vi "TCP单点接收.main.vi"(0 "IP地址":string="127.0.0.1" caption="服务名称", 1 "端口号":i32=6314, 2 "储存路径":path=path "D:/AA", 5 "error IO":errorcluster caption="错误输入") -> (14 "已收百分比":string, 15 "运行指示灯":bool, 19 "错误输出 2":errorcluster caption="错误输出")   [LabVIEW 2016, in "TCP文件传输系统.lvlib" / "TCP接收文件.lvlib"]
panel:
  in  "分一包（兆）":i64=40
  out "文件名":string
  out "2":errorcluster caption="错误输出"
  out "单包大小":i32
  out "帧数":i32
  out "帧号":i32
  out "错误输出":errorcluster
  out "路径 2":path
  out "已收次数":i32
  out "需接收次数":i32
  in  "停止 2":bool
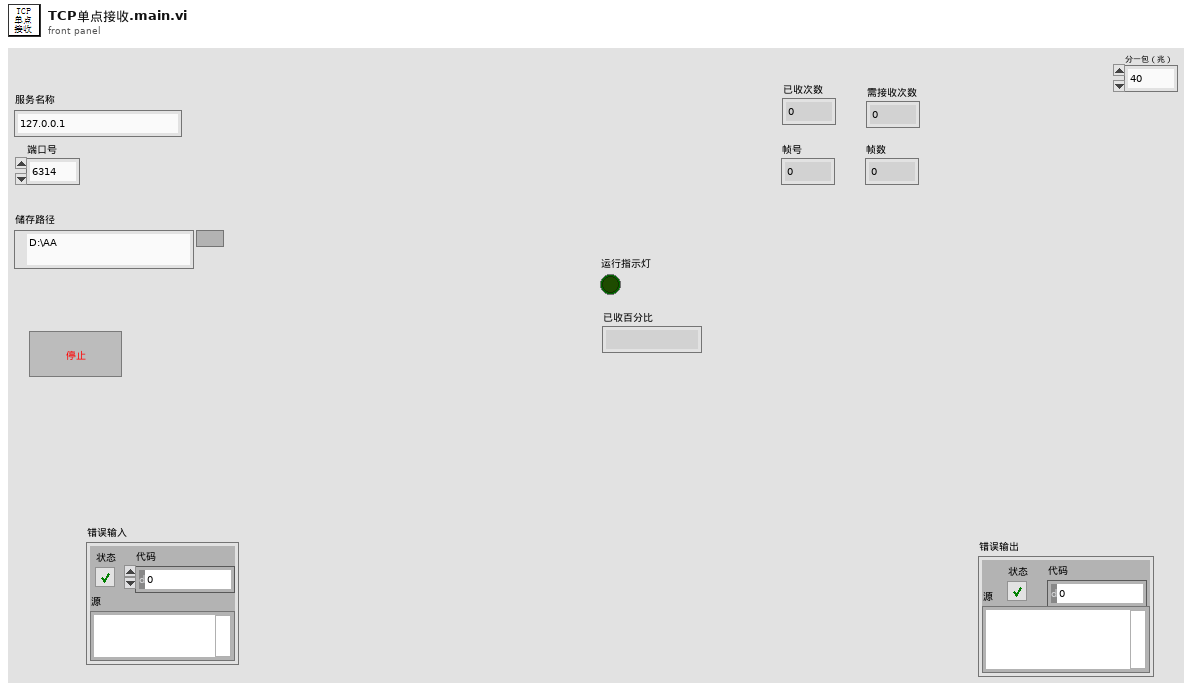
[diagram p1: front panel]
types:
  T1 = cluster{"网络灯":bool, "接收中":bool, "已接收百分比":string, "接收成功次数":dbl}
  T2 = enum16{"open", "replace", "create", "open or create", "replace or create", "replace or create with confirmation"}
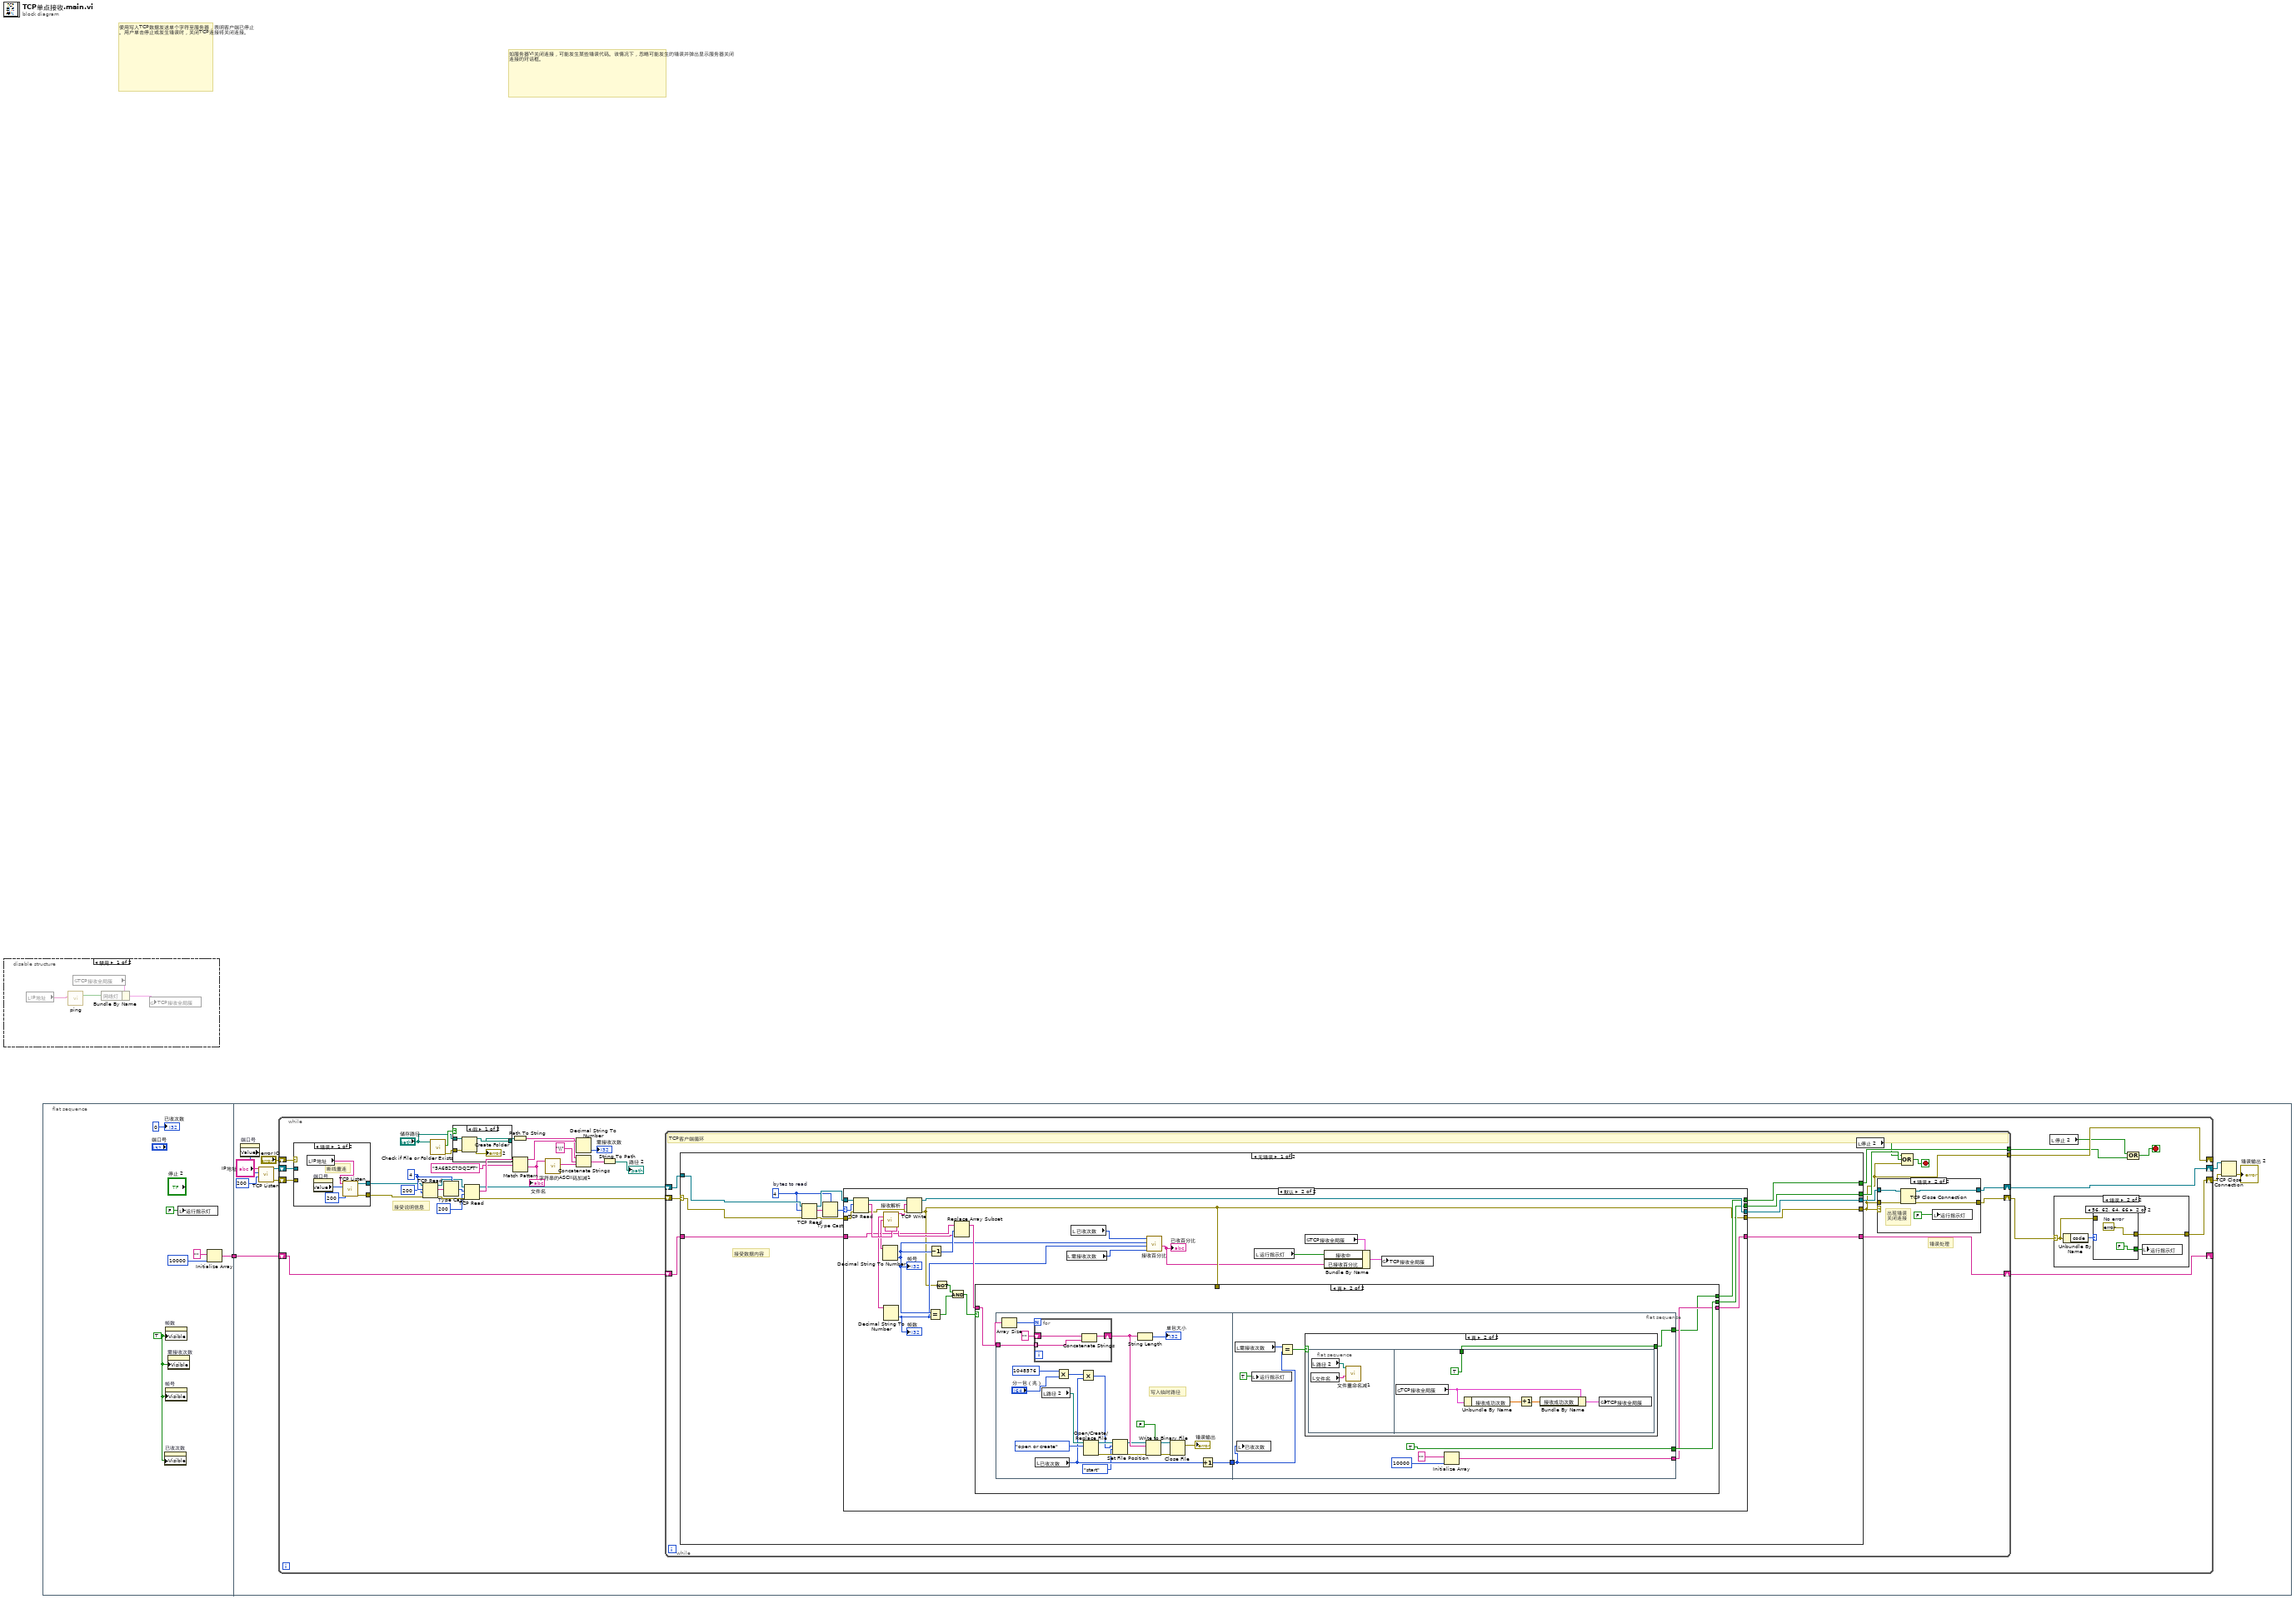
[diagram p0: block diagram]
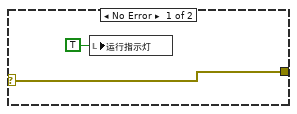
[diagram p3: hidden frame]
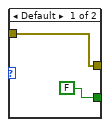
[diagram p4: hidden frame]
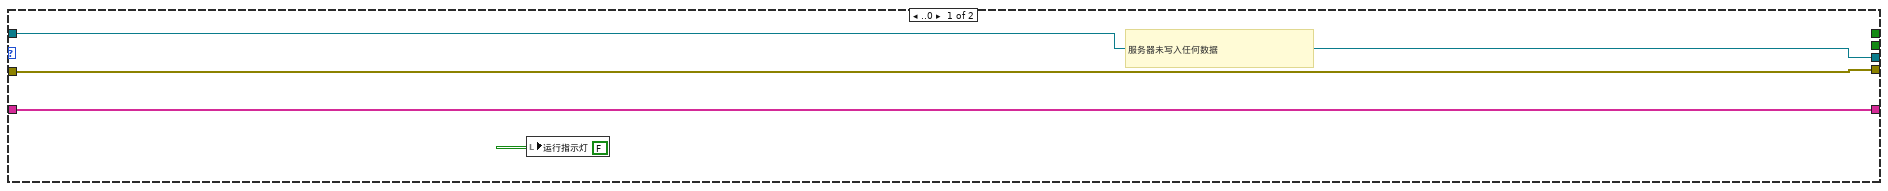
[diagram p8: hidden frame]
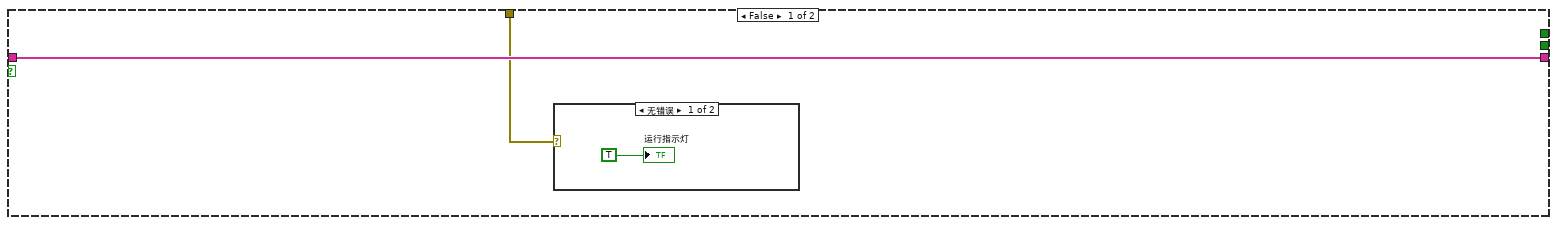
[diagram p9: hidden frame]
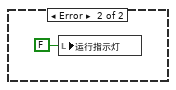
[diagram p10: hidden frame]
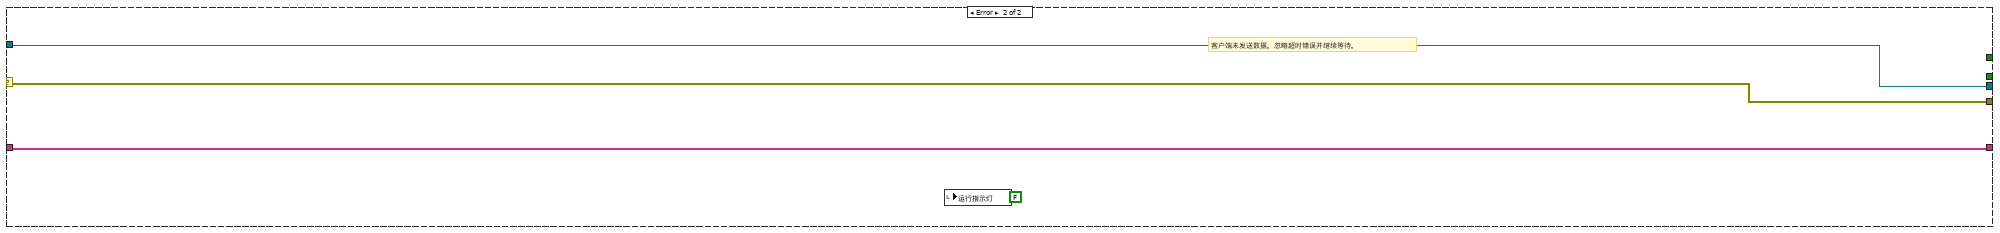
[diagram p12: hidden frame]
diagram:
  # "如服务器VI关闭连接，可能发生某些错误代码。该情况下，忽略可能发生的错误并弹出显示服务器关闭连接的对话框。"
  # "使用写入TCP数据发送单个字符至服务器，表明客户端已停止。用户单击停止或发生错误时，关闭TCP连接将关闭连接。"
  n1 = disable-structure shown="禁用" {
    frame Disabled {
      n2 = local read "IP地址"() -> (w5:string)
      n3 = call "ping.vi"("IP"=w5) -> ("ping结果"=w2:bool)  [unwired: 10 in]
      n4 = global read "全局变量1.vi" "TCP接收全局簇"() -> (w3:T1)
      n5 = Bundle By Name(cluster=w3, "网络灯"=w2) -> (w4:T1)
      n6 = global write "全局变量1.vi" "TCP接收全局簇"(w4) -> ()
    }
    frame Enabled {
    }
  }
  n7 = flat-sequence {
    tunnel: [w8] -> w1
    tunnel: w1 -> [w21]
    frame #0 {
      w7 = TRUE ("可见")
      n8 = property on="已收次数" class="DigNum (严格)"("Visible"=w7) -> ()  [unwired: 2 in, 2 out]
      n9 = property on="帧数" class="DigNum (严格)"("Visible"=w7) -> ()  [unwired: 2 in, 2 out]
      n10 = property on="帧号" class="DigNum (严格)"("Visible"=w7) -> ()  [unwired: 2 in, 2 out]
      n11 = property on="需接收次数" class="DigNum (严格)"("Visible"=w7) -> ()  [unwired: 2 in, 2 out]
      n12 = local write "运行指示灯"(FALSE ("运行指示灯")) -> ()
      n13 = Initialize Array("", 10000 ("维数大小")) -> (w8:string[])
      "已收次数" <- i64 0 ("已发次数")
    }
    frame #1 {
      n14 = property on="端口号" class="DigNum (严格)"() -> ("Value"=w15:i32)  [unwired: 2 in, 2 out]
      n15 = call <vilib>:"TCP Listen.vi"("timeout ms (wait forever: -1)"=200, "port"=w15, "service name"="IP地址") -> ("error out"=w20:errorcluster, "connection ID"=w19:refnum<k5>)  [unwired: 4 in, 3 out]
      n16 = while {
        shift-right: [w44] -> _
        shift-left: w21 -> [w43]
        shift-right: [w58] -> w17
        shift-left: w19 -> [w42]
        shift-right: [w28] -> w18
        shift-left: w20 -> [w41]
        shift-right: [w39] -> _
        shift-left: "error IO" -> [w38]
        stop <- w22 stop-if-true
        w57 = 4 ("读取的字节")
        # "接受说明信息"
        n17 = case shown="错误" w38 {
          tunnel: w42 -> [_ w80]
          tunnel: [w78 w80] -> w27
          tunnel: w41 -> [_ w79]
          tunnel: [w77 w79] -> w26
          frame Error {
            # "断线重连"
            n18 = local read "IP地址"() -> (w74:string)
            n19 = property on="端口号" class="DigNum (严格)"() -> ("Value"=w75:i32)  [unwired: 2 in, 2 out]
            n20 = call <vilib>:"TCP Listen.vi"("timeout ms (wait forever: -1)"=200, "port"=w75, "service name"=w74) -> ("error out"=w77:errorcluster, "connection ID"=w78:refnum<k5>)  [unwired: 4 in, 3 out]
          }
          frame No Error {
          }
        }
        n21 = TCP Read(connection ID=w27, bytes to read=w57, error in (no error)=w26, 9:200 ("超时毫秒(25000)")) -> (connection ID out=w53:refnum<k5>, data out=w56:string, error out=w54:errorcluster)  [unwired: 1 in]
        n22 = call <vilib>:"Check if File or Folder Exists.vi"("path"="储存路径") -> ("error out"=w36:errorcluster, "file or folder exists?"=w37:bool)  [unwired: 8 in, 1 out]
        n23 = Type Cast(type=w57, x=w56) -> (*(type *) &x=w55:i32)
        n24 = case shown="假" w37 {
          tunnel: "储存路径" -> [w72 w73]
          tunnel: w36 -> [w71 _]
          tunnel: [w70 w73] -> w33
          frame False {
            n25 = Create Folder(path (use dialog)=w72, error in=w71) -> (created path=w70:path, error out=→"2":errorcluster)  [unwired: 1 in, 1 out]
          }
          frame True {
          }
        }
        n26 = TCP Read(connection ID=w53, bytes to read=w55, error in (no error)=w54, 9:200 ("超时毫秒(25000)")) -> (connection ID out=w40:refnum<k5>, data out=w52:string, error out=w30:errorcluster)  [unwired: 1 in]
        n27 = Path To String(path=w33) -> (string=w34:string)
        n28 = Match Pattern(string=w52, regular expression="5A6B2C7DQZFT" ("正则表达式")) -> (before substring=w50:string, after substring=w32:string)  [unwired: 1 in, 2 out]
        "文件名" <- w32
        n29 = call "字符串的ASCII码加减1.vi"("原字符串"=w32) -> ("ASCII码"=w31:string)  [unwired: 10 in]
        n30 = Decimal String To Number(string=w50) -> (number=→"需接收次数":i32)  [unwired: 2 in, 1 out]
        n31 = Concatenate Strings(w34, "\\" ("字符串"), w31) -> (w48:string)
        n32 = String To Path(string=w48) -> (path=→"路径 2":path)
        n33 = while {
          tunnel: [w89] -> w23
          shift-right: [w88] -> w44
          shift-left: w43 -> [w87]
          shift-right: [w82] -> w29
          shift-left: w30 -> [w91]
          shift-right: [w85] -> w58
          shift-left: w40 -> [w84]
          tunnel: [w83] -> w39
          stop <- w92 stop-if-true
          # "错误处理"
          # "TCP客户端循环"
          n34 = case shown="无错误" w91 {
            selector: w91 -> [w111 w199]
            tunnel: [w110 w199] -> w83
            tunnel: w84 -> [w112 w200]
            tunnel: [w109 w200] -> w86
            tunnel: [w108 _] -> w90
            tunnel: [w107 _] -> w89
            tunnel: [w106 w198] -> w88
            tunnel: w87 -> [w105 w198]
            frame No Error {
              w102 = 4  # bytes to read
              # "接受数据内容"
              n35 = TCP Read(connection ID=w112, bytes to read=w102, error in (no error)=w111) -> (connection ID out=w104:refnum<k5>, data out=w100:string, error out=w103:errorcluster)  [unwired: 2 in]
              n36 = Type Cast(type=w102, x=w100) -> (*(type *) &x=w101:i32)
              n37 = case shown="默认" w101 {
                selector: w101 -> [_ w143]
                tunnel: w104 -> [w116 w145]
                tunnel: w103 -> [w115 w144]
                tunnel: [w116 w137] -> w109
                tunnel: [w115 w121] -> w110
                tunnel: [_ w135] -> w108
                tunnel: [_ w132] -> w107
                tunnel: [w114 w129] -> w106
                tunnel: w105 -> [w114 w130]
                frame ..0 {
                  # "服务器未写入任何数据"
                  n38 = local write "运行指示灯"(FALSE ("运行指示灯")) -> ()
                }
                frame Default {
                  n39 = TCP Read(connection ID=w145, bytes to read=w143, error in (no error)=w144) -> (connection ID out=w139:refnum<k5>, data out=w142:string, error out=w138:errorcluster)  [unwired: 2 in]
                  n40 = call "接收解析.vi"("data in"=w142) -> ("重算CRC32"=w134:string, "帧数"=w136:string, "帧号"=w141:string, "帧内容"=w133:string)  [unwired: 3 in, 8 out]
                  n41 = Decimal String To Number(string=w141) -> (number=w126:i32)  [unwired: 2 in, 1 out]
                  "帧号" <- w126
                  n42 = Decimal String To Number(string=w136) -> (number=w125:i32)  [unwired: 2 in, 1 out]
                  "帧数" <- w125
                  n43 = TCP Write(connection ID=w139, data in=w134, error in (no error)=w138) -> (connection ID out=w137:refnum<k5>, error out=w121:errorcluster)  [unwired: 1 in, 1 out]
                  n44 = Equal?(x=w126, y=w125) -> (x = y?=w124:bool)
                  n45 = Decrement(x=w126) -> (x-1=w140:i32)
                  n46 = Not(x=w121) -> (.not. x?=w123:bool)
                  n47 = And(x=w123, y=w124) -> (x .and. y?=w122:bool)
                  n48 = Replace Array Subset(array=w130, new element=w133, index=w140) -> (w131:string[])
                  n49 = case shown="真" w122 {
                    tunnel: [_ w153] -> w135
                    tunnel: w131 -> [w147 w154]
                    tunnel: [_ w150] -> w132
                    tunnel: [w147 w151] -> w129
                    tunnel: w121 -> [w146 _]
                    frame False {
                      n50 = case shown="无错误" w146 {
                        frame No Error {
                          "运行指示灯" <- TRUE ("运行指示灯")
                        }
                        frame Error {
                          n51 = local write "运行指示灯"(FALSE ("运行指示灯")) -> ()
                        }
                      }
                    }
                    frame True {
                      n52 = flat-sequence {
                        tunnel: w154 -> [w167]
                        tunnel: [w175] -> w152
                        tunnel: [TRUE] -> w153
                        tunnel: w152 -> [w187]
                        tunnel: [w184] -> w150
                        tunnel: [w181] -> w151
                        frame #0 {
                          # "写入临时路径"
                          n53 = Array Size(array=w167) -> (size(s)=w168:i32)
                          n54 = for {
                            N: w168 -> [_]
                            shift-right: [w179] -> w166
                            shift-left: "" -> [w178]
                            tunnel: w167 -> [w177] mode=indexing
                            n55 = Concatenate Strings(w178, w177) -> (w179:string)
                          }
                          n56 = local read "已收次数"() -> (w160:i32)
                          n57 = local read "路径 2"() -> (w176:path)
                          n58 = Multiply(x=i64 1048576, y="分一包（兆）") -> (x*y=w156:i64)
                          n59 = Multiply(x=w156, y=w160) -> (x*y=w159:i64)
                          n60 = Open/Create/Replace File(file path (use dialog)=w176, operation (0:open)=T2."open or create" ("操作(0:open)")) -> (refnum out=w163:refnum<file>, error out=w164:errorcluster)  [unwired: 4 in, 1 out]
                          n61 = Set File Position(offset (in bytes) (0)=w159, refnum=w163, from (0:start)=enum16{"start", "end", "current"}."start" ("自（0:起始）"), error in=w164) -> (refnum out=w161:refnum<file>, error out=w162:errorcluster)
                          n62 = String Length(string=w166) -> (length=→"单包大小":i32)
                          n63 = Write to Binary File(file (use dialog)=w161, data=w166, error in=w162, 5:FALSE ("预置数组或字符串大小？(T)")) -> (refnum out=w173:refnum<file>, error out=w174:errorcluster)  [unwired: 2 in, 1 out]
                          n64 = Close File(refnum=w173, error in=w174) -> (error out=→"错误输出":errorcluster)  [unwired: 1 out]
                          n65 = Increment(x=w160) -> (x+1=w175:i32)
                        }
                        frame #1 {
                          n66 = local read "需接收次数"() -> (w186:i32)
                          n67 = local write "已收次数"(w187) -> ()
                          n68 = local write "运行指示灯"(TRUE ("运行指示灯")) -> ()
                          n69 = Equal?(x=w186, y=w187) -> (x = y?=w185:bool)
                          n70 = case shown="真" w185 {
                            tunnel: [_ w189] -> w184
                            frame False {
                            }
                            frame True {
                              n71 = flat-sequence {
                                tunnel: [TRUE] -> w189
                                frame #0 {
                                n72 = local read "文件名"() -> (w190:string)
                                n73 = local read "路径 2"() -> (w191:path)
                                n74 = call "文件重命名减1.vi"("名称或相对路径"=w190, "源路径"=w191) -> ()  [unwired: 10 in]
                                }
                                frame #1 {
                                n75 = global read "全局变量1.vi" "TCP接收全局簇"() -> (w192:T1)
                                n76 = Unbundle By Name(w192) -> ("接收成功次数"=w193:dbl)
                                n77 = Increment(x=w193) -> (x+1=w194:dbl)
                                n78 = Bundle By Name(cluster=w192, "接收成功次数"=w194) -> (w195:T1)
                                n79 = global write "全局变量1.vi" "TCP接收全局簇"(w195) -> ()
                                }
                              }
                            }
                          }
                          n80 = Initialize Array("", 10000 ("维数大小")) -> (w181:string[])
                        }
                      }
                    }
                  }
                  n81 = local read "需接收次数"() -> (w127:i32)
                  n82 = local read "已收次数"() -> (w128:i32)
                  n83 = call "接收百分比.vi"("需发送次数"=w127, "帧数"=w125, "帧号"=w126, "已收次数"=w128) -> ("已收百分比"=w118:string)  [unwired: 7 in]
                  "已收百分比" <- w118
                  n84 = local read "运行指示灯"() -> (w117:bool)
                  n85 = global read "全局变量1.vi" "TCP接收全局簇"() -> (w119:T1)
                  n86 = Bundle By Name(cluster=w119, "接收中"=w117, "已接收百分比"=w118) -> (w120:T1)
                  n87 = global write "全局变量1.vi" "TCP接收全局簇"(w120) -> ()
                }
              }
            }
            frame Error {
              # "客户端未发送数据。忽略超时错误并继续等待。"
              n88 = local write "运行指示灯"(FALSE ("运行指示灯")) -> ()
            }
          }
          n89 = local read "停止 2"() -> (w81:bool)
          n90 = case shown="错误" w83 {
            tunnel: [w94 w97] -> w82
            tunnel: w83 -> [w94 w98]
            tunnel: [w93 w96] -> w85
            tunnel: w86 -> [w93 w99]
            frame No Error {
            }
            frame Error {
              # "出现错误\n关闭连接"
              n91 = TCP Close Connection(connection ID=w99, error in (no error)=w98) -> (connection ID out=w96:refnum<k5>, error out=w97:errorcluster)  [unwired: 1 in]
              n92 = local write "运行指示灯"(FALSE ("运行指示灯")) -> ()
            }
          }
          n93 = Compound Arithmetic op=OR(w81, w90, w83) -> (w92:bool)
        }
        n94 = local read "停止 2"() -> (w24:bool)
        n95 = case shown="错误" w29 {
          selector: w29 -> [w60 w63]
          tunnel: [w60 w62] -> w28
          frame No Error {
            n96 = local write "运行指示灯"(TRUE ("运行指示灯")) -> ()
          }
          frame Error {
            n97 = Unbundle By Name(w63) -> ("code"=w64:i32)
            n98 = case shown="56, 62, 64, 66" w64 {
              tunnel: w63 -> [w66 _]
              tunnel: [w66 w68] -> w62
              tunnel: [FALSE FALSE] -> w61
              frame Default {
              }
              frame 56, 62, 64, 66 {
                w68 = errorcluster {"status"=FALSE, "code"=0, "source"=""}  # No error
              }
            }
            n99 = local write "运行指示灯"(w61) -> ()
          }
        }
        n100 = Compound Arithmetic op=OR(w24, w23) -> (w22:bool)
      }
      n101 = TCP Close Connection(connection ID=w17, error in (no error)=w18) -> (error out=→"错误输出 2":errorcluster)  [unwired: 1 in, 1 out]
    }
  }
